vi "Are Equal.vi"(8 "error in":errorcluster, 9 "Received Text":string, 10 "Approved Text":string, 11 "JSON Comparator in":refnum<class "JSON Comparator.lvclass">) -> (0 "error out":errorcluster, 2 "Are Equal?":bool, 3 "JSON Comparator out":refnum<class "JSON Comparator.lvclass">)   [LabVIEW 2020, in "Approval Tests.lvlib" / "JSON Comparator.lvclass"]
uses:
  JSON Comparator.lvclass
  <vilib>/JDP Science/JSONtext/JSONtext.lvlib
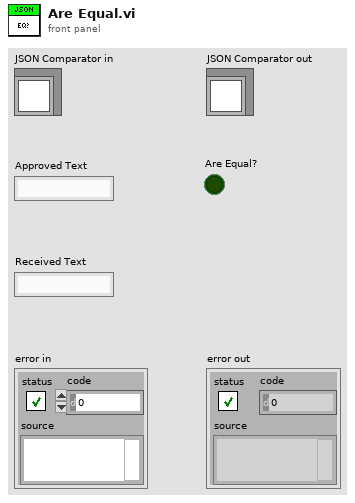
[diagram p1: front panel]
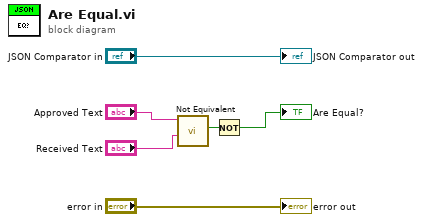
[diagram p0: block diagram]
diagram:
  n1 = call <vilib>:"Not Equivalent.vi"("Other JSON"="Received Text", "JSON"="Approved Text") -> ("Not Equivalent"=w2:bool)  [unwired: 8 in]
  n2 = Not(x=w2) -> (.not. x?=→"Are Equal?":bool)
  "error out" <- "error in"
  "JSON Comparator out" <- "JSON Comparator in"
